vi "LowerArmFlip.vi"(6 "Degree to which\n its lowered":dbl, 8 "error in":errorcluster, 9 "FPGA VI Reference In":T1, 10 "milliseconds to wait \nfor servo to change":u32=100, 11 "Old Angle":dbl) -> (0 "error out":errorcluster, 1 "FPGA VI Reference Out":T1, 2 "milliseconds to wait \nfor servo to change Out":u32, 3 "New Angle":dbl)   [LabVIEW 2012]
uses:
  FPGA_ref.ctl
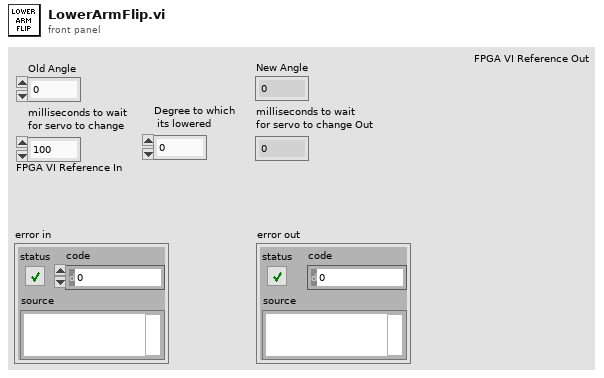
[diagram p1: front panel]
types:
  T1 = typedef "FPGA_ref.ctl" = refnum<k20>
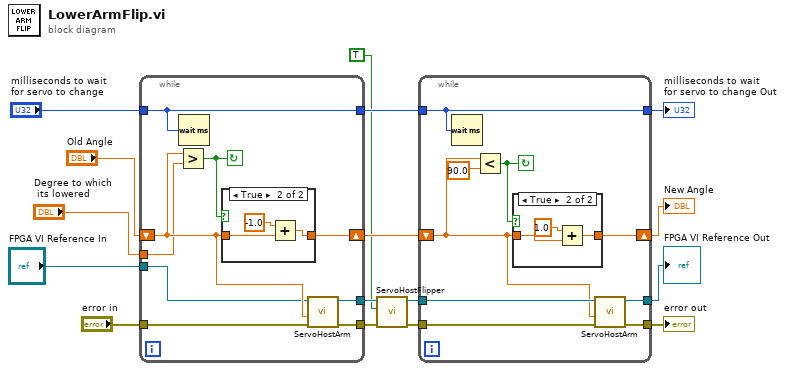
[diagram p0: block diagram]
diagram:
  n1 = while {
    tunnel: "error in" -> [w20]
    shift-right: [w24] -> w7
    shift-left: "Old Angle" -> [w21]
    tunnel: "milliseconds to wait \nfor servo to change" -> [w23]
    tunnel: [w23] -> w8
    tunnel: [w22] -> w4
    tunnel: "FPGA VI Reference In" -> [w19]
    tunnel: [w18] -> w5
    tunnel: "Degree to which\n its lowered" -> [w17]
    stop <- w25 continue-if-true
    n2 = Greater?(x=w21, y=w17) -> (0:w25:bool)
    n3 = Wait (ms)(milliseconds to wait=w23) -> ()  [unwired: 1 out]
    n4 = case shown="True" w25 {
      tunnel: w21 -> [w26 w29]
      tunnel: [w26 w27] -> w24
      frame False {
      }
      frame True {
        n5 = Add(x=-1.0, y=w29) -> (x+y=w27:dbl)
      }
    }
    n6 = call "ServoHostArm.vi"("error in"=w20, "Angle (deg) Arm"=w21, "FPGA VI Reference In"=w19) -> ("error out"=w22:errorcluster, "FPGA VI Reference Out 2"=w18:T1)  [unwired: 7 in]
  }
  n7 = call "ServoHostFlipper.vi"("error in"=w4, "Hi/Lo"=TRUE, "FPGA VI Reference In"=w5) -> ("error out"=w3:errorcluster, "FPGA VI Reference Out"=w6:T1)  [unwired: 7 in]
  n8 = while {
    tunnel: w3 -> [w35]
    shift-right: [w38] -> w9
    shift-left: w7 -> [w32]
    tunnel: w8 -> [w37]
    tunnel: [w37] -> w10
    tunnel: [w36] -> w11
    tunnel: w6 -> [w34]
    tunnel: [w33] -> w12
    stop <- w31 continue-if-true
    n9 = Wait (ms)(milliseconds to wait=w37) -> ()  [unwired: 1 out]
    n10 = Less?(x=w32, y=90.0) -> (x < y?=w31:bool)
    n11 = case shown="True" w31 {
      tunnel: w32 -> [w39 w42]
      tunnel: [w39 w40] -> w38
      frame False {
      }
      frame True {
        n12 = Add(x=1.0, y=w42) -> (x+y=w40:dbl)
      }
    }
    n13 = call "ServoHostArm.vi"("error in"=w35, "Angle (deg) Arm"=w32, "FPGA VI Reference In"=w34) -> ("error out"=w36:errorcluster, "FPGA VI Reference Out 2"=w33:T1)  [unwired: 7 in]
  }
  "New Angle" <- w9
  "error out" <- w11
  "milliseconds to wait \nfor servo to change Out" <- w10
  "FPGA VI Reference Out" <- w12
